vi "Error Message.vi"() -> (2 "Error":string)   [LabVIEW 2015]
uses:
  Galobal variable_TI.vi
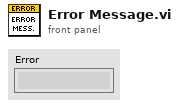
[diagram p1: front panel]
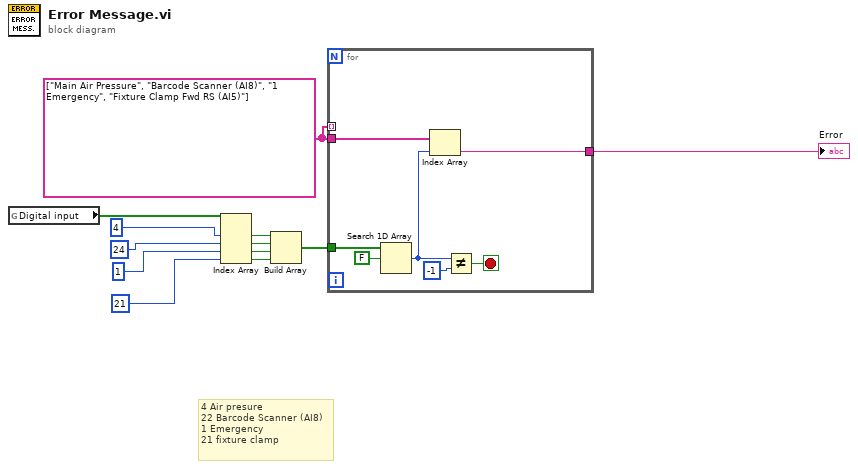
[diagram p0: block diagram]
diagram:
  w5 = string[] ["Main Air Pressure", "Barcode Scanner (AI8)", "1 Emergency", "Fixture Clamp Fwd RS (AI5)"]
  # "4 Air presure\n22 Barcode Scanner (AI8)\n1 Emergency\n21 fixture clamp"
  n1 = global read "Galobal variable_TI.vi" "Digital input"() -> (w12:bool[])
  n2 = Index Array(array=w12, index #1=4 ("index"), index #2=24 ("index"), index #3=1 ("index"), index #4=21 ("index")) -> (element #1=w8:bool, element #2=w7:bool, element #3=w6:bool, element #4=w1:bool)
  n3 = Build Array(w8, w7, w6, w1) -> (w4:bool[])
  n4 = for {
    tunnel: w5 -> [_] mode=indexing
    tunnel: w5 -> [w15]
    tunnel: w4 -> [w17]
    tunnel: [w13] -> w3
    stop <- w16 stop-if-true
    n5 = Search 1D Array(1D array=w17, element=FALSE) -> (index of element=w14:i32)  [unwired: 1 in]
    n6 = Index Array(array=w15, index=w14) -> (element=w13:string)
    n7 = Not Equal?(x=w14, y=-1) -> (x != y?=w16:bool)
  }
  "Error" <- w3
